vi "cam_track.vi"(6 "Trigger":bool, 7 "state change":bool, 8 "gun_rt_slow_downstream_data out in":T3, 9 "gun_rt_fast_downstream_data out":T4, 11 "Gains":T1) -> (2 "Lock":bool, 3 "gun_rt_slow_downstream_data out out":T3)   [LabVIEW 2011]
uses:
  gun_rt_slow_downstream_data.ctl
  gun_rt_fast_downstream_data.ctl
  gun_motor_state.ctl
  common/scale_const.ctl
  common/gain_bin_sched_const.ctl
  signals/Signal.ctl
  2012vision/Camera State.ctl
panel:
  in  "lock const":dbl=4.0
  in  "invert gains":bool
  out "settle time":dbl
  in  "Integral Cap":T2={"min_ana"=0.0, "min_units"=0.6, "max_ana"=0.4, "max_units"=0.0}
  in  "stop_track_time":u32=200
  in  "Cam Jitter Time":u32=500
  in  "Reset Integral":bool
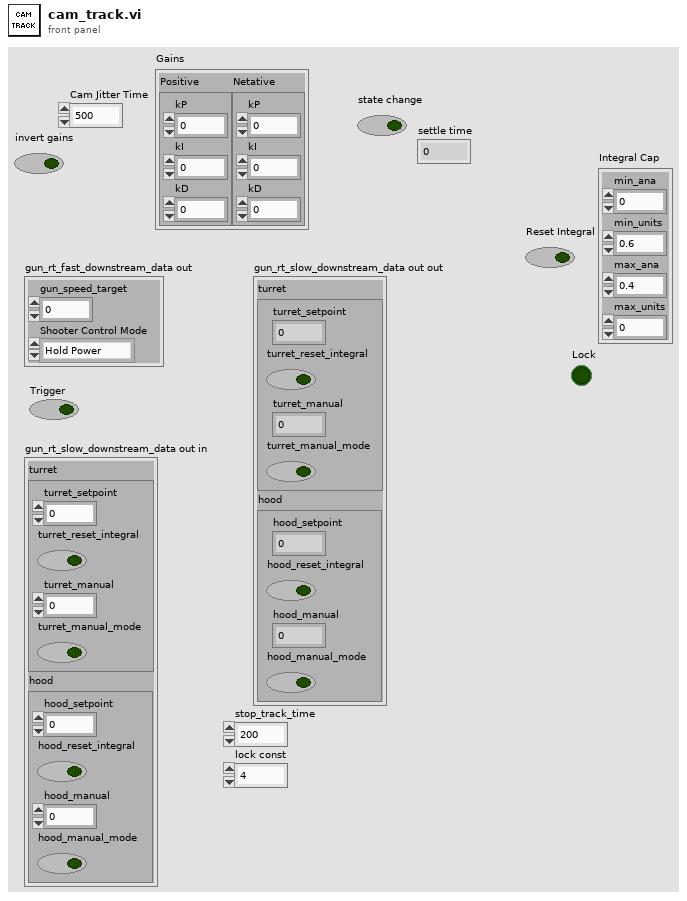
[diagram p1: front panel]
types:
  T1 = typedef "gain_bin_sched_const.ctl" = cluster{"Positive":cluster{"kP":dbl, "kI":dbl, "kD":dbl}, "Netative":cluster{"kP":dbl, "kI":dbl, "kD":dbl}}
  T2 = typedef "scale_const.ctl" = cluster{"min_ana":dbl, "min_units":dbl, "max_ana":dbl, "max_units":dbl}
  T3 = typedef "gun_rt_slow_downstream_data.ctl" = cluster{"turret":cluster{"turret_setpoint":dbl, "turret_reset_integral":bool, "turret_manual":dbl, "turret_manual_mode":bool}, "hood":cluster{"hood_setpoint":dbl, "hood_reset_integral":bool, "hood_manual":dbl, "hood_manual_mode":bool}}
  T4 = typedef "gun_rt_fast_downstream_data.ctl" = cluster{"gun_speed_target":dbl, "Shooter Control Mode":T5}
  T5 = typedef "gun_motor_state.ctl" = enum16{"Hold Power", "Hold Speed", "Hold Distance", "Stop"}
  T6 = typedef "Signal.ctl" = enum16{"SIGFIRE", "SIGSTOPSCRIPT", "SIGSTARTGUN", "SIGSTOPGUN", "SIGDISABLED", "SIGENABLED", "SIGUDPTIMEOUT", "SIGNEWVISION_REMOTE", "SIGNEWVISION_LOCAL", "SIGSHOTFIRED", "SIGDOTRACK", "SIGDONTTRACK"}
  T7 = typedef "Camera State.ctl" = enum16{"No Targets", "Low Confidence", "Medium Confidence", "High Confidence", "Camera Error"}
  T8 = enum16{"Get Latest Data", "Get Local Data", "Get Remote Data", "Set Local Data", "Set Remote Data"}
  T9 = cluster{"X Position":dbl, "Distance":dbl, "Camera State":T7}
  T10 = typedef "gain_const.ctl" = cluster{"kP":dbl, "kI":dbl, "kD":dbl}
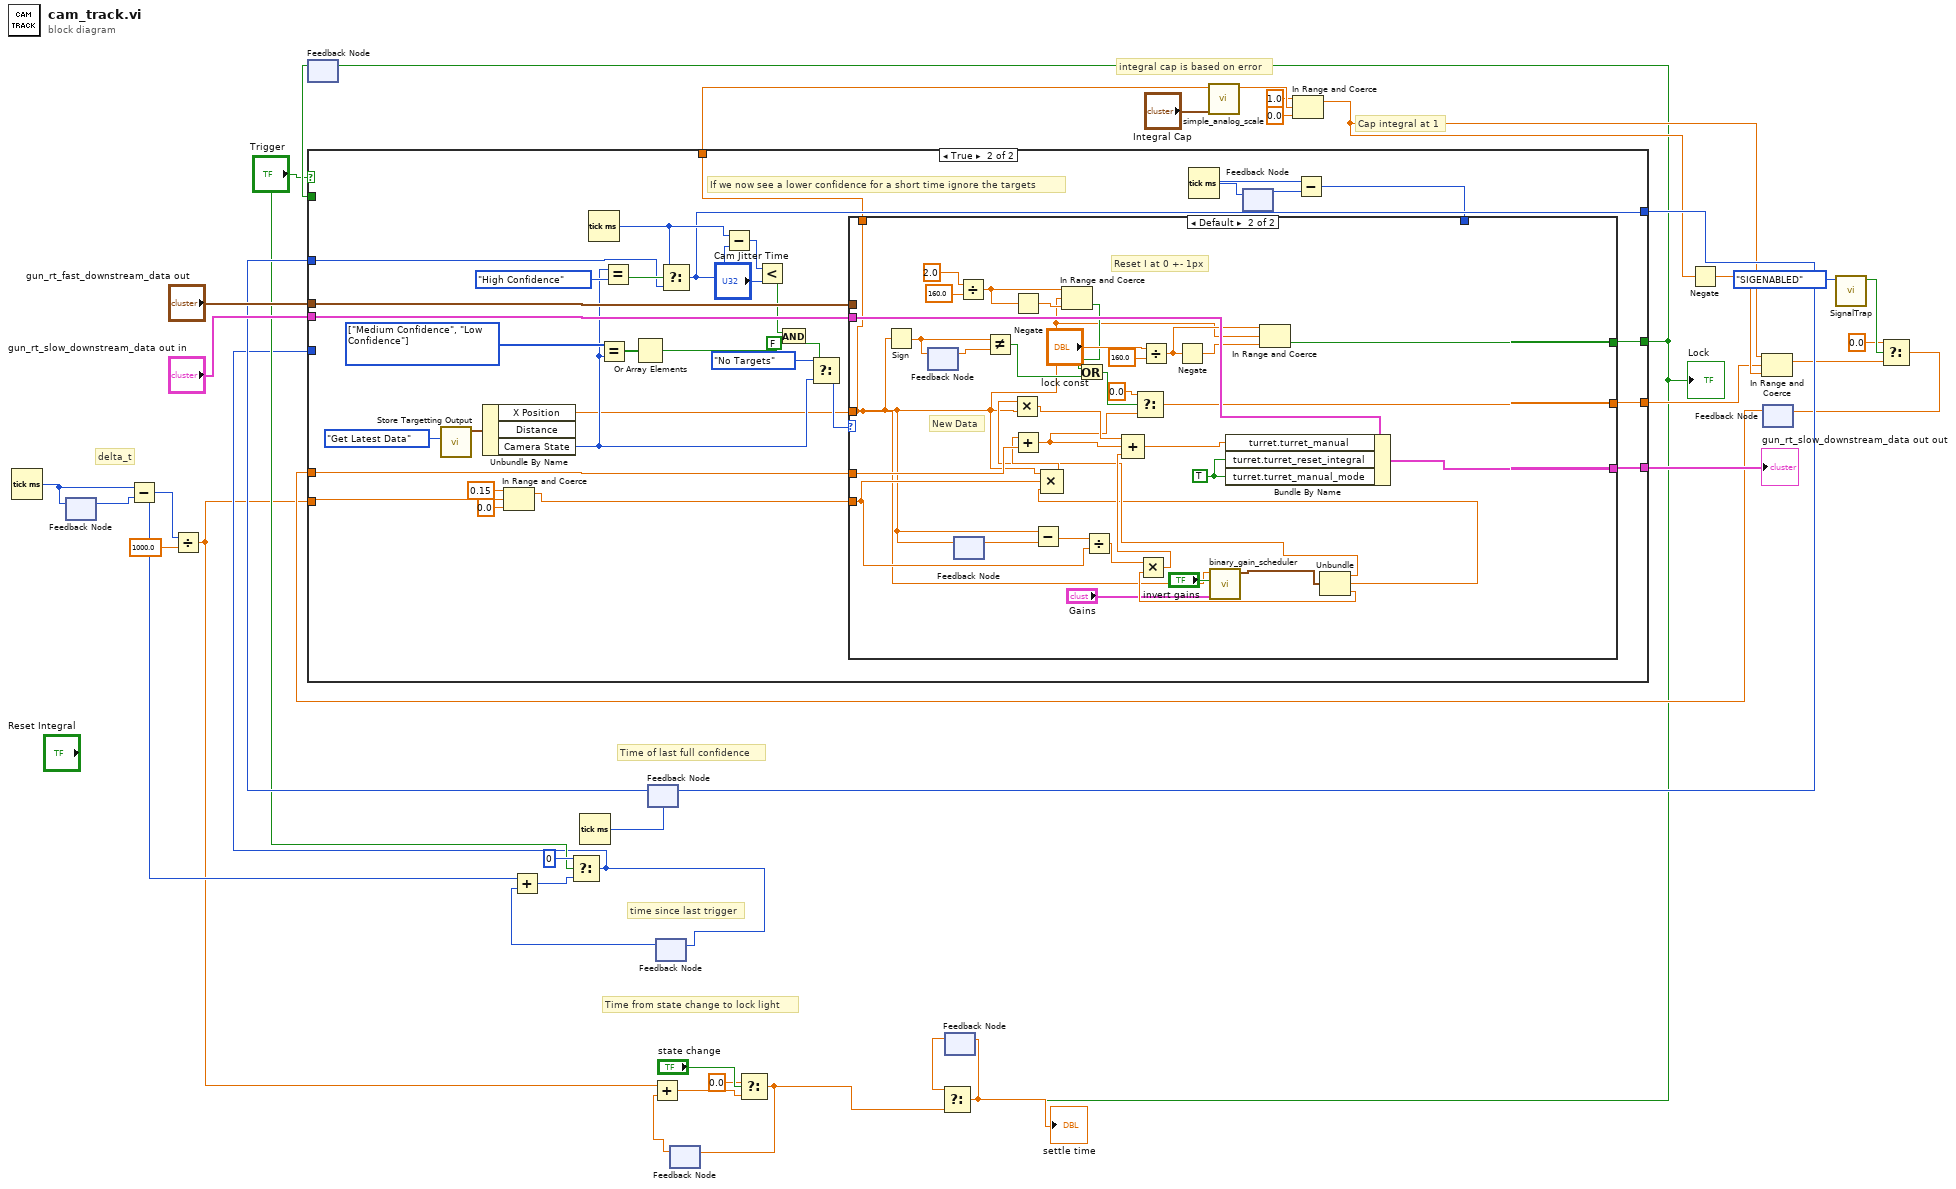
[diagram p0: block diagram]
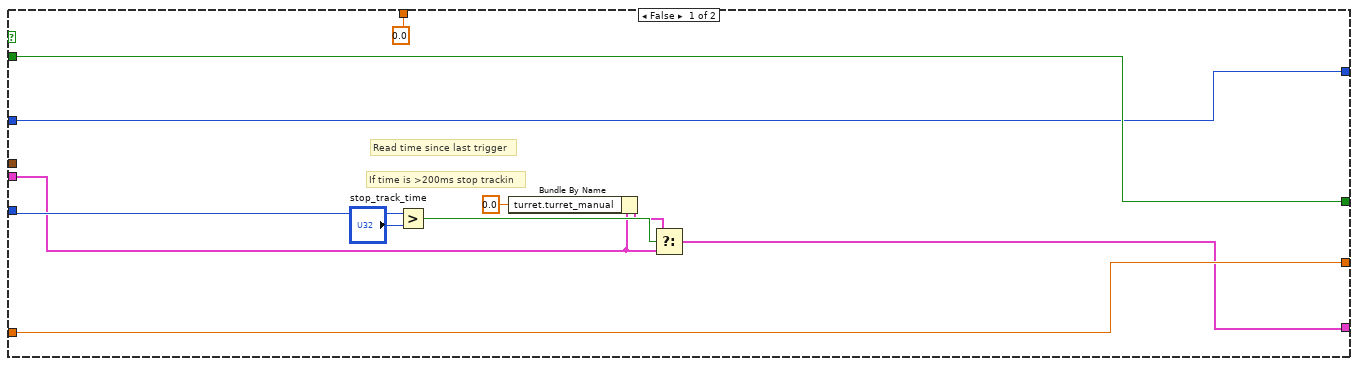
[diagram p2: hidden frame]
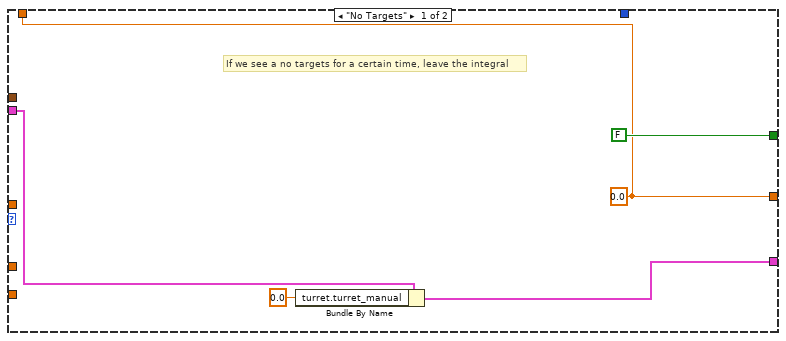
[diagram p3: hidden frame]
diagram:
  # "Time from state change to lock light"
  # "integral cap is based on error"
  # "time since last trigger"
  # "delta_t"
  # "Time of last full confidence"
  # "Cap integral at 1"
  n1 = Tick Count (ms)() -> (millisecond timer value=w30:u32)
  n2 = feedback-in #1(w30) -> ()
  n3 = feedback #1() -> (w29:u32)  [unwired: 1 in]
  n4 = Subtract(x=w30, y=w29) -> (x-y=w15:u32)
  n5 = Divide(x=w15, y=1000.0) -> (x/y=w9:dbl)
  n6 = feedback #2() -> (w36:bool)  [unwired: 1 in]
  n7 = Tick Count (ms)() -> (millisecond timer value=w33:u32)
  n8 = feedback #3(w33) -> (w32:u32)
  n9 = feedback #4() -> (w28:u32)  [unwired: 1 in]
  n10 = Add(x=w15, y=w28) -> (x+y=w27:u32)
  n11 = Select(t=u32 0, s="Trigger", f=w27) -> (s? t:f=w24:u32)
  n12 = feedback-in #4(w24) -> ()
  n13 = feedback #5() -> (w14:dbl)  [unwired: 1 in]
  n14 = Add(x=w9, y=w14) -> (x+y=w13:dbl)
  n15 = Select(t=0.0, s="state change", f=w13) -> (s? t:f=w1:dbl)
  n16 = feedback-in #5(w1) -> ()
  n17 = feedback #6() -> (w2:dbl)  [unwired: 1 in]
  n18 = feedback #7() -> (w35:dbl)  [unwired: 1 in]
  n19 = case shown="True" "Trigger" {
    tunnel: "gun_rt_slow_downstream_data out in" -> [w42 w80]
    tunnel: "gun_rt_fast_downstream_data out" -> [_ w79]
    tunnel: [w44 w78] -> w39
    tunnel: w36 -> [w50 _]
    tunnel: [w50 w77] -> w3
    tunnel: w35 -> [w49 w75]
    tunnel: [w49 w76] -> w16
    tunnel: w32 -> [w48 w72]
    tunnel: [w48 w67] -> w31
    tunnel: w24 -> [w47 _]
    tunnel: w9 -> [_ w57]
    tunnel: [0.0 ("X Position") w59] -> w22
    frame False {
      # "If time is >200ms stop trackin"
      # "Read time since last trigger"
      n20 = Greater?(x=w47, y="stop_track_time") -> (0:w45:bool)
      n21 = Bundle By Name(cluster=w42, "turret.turret_manual"=0.0) -> (w43:T3)
      n22 = Select(t=w43, s=w45, f=w42) -> (s? t:f=w44:T3)
    }
    frame True {
      w71 = T7[] [enum."Medium Confidence", enum."Low Confidence"] items=["No Targets", "Low Confidence", "Medium Confidence", "High Confidence", "Camera Error"]
      # "If we now see a lower confidence for a short time ignore the targets"
      n23 = call "Store Targetting Output.vi"("mode"=T8."Get Latest Data") -> ("Targetting Output"=w81:T9)  [unwired: 10 in]
      n24 = Unbundle By Name(w81) -> ("X Position"=w60:dbl, "Camera State"=w63:T7)  [unwired: 1 out]
      n25 = In Range and Coerce(upper limit=0.15, x=w57, lower limit=0.0) -> (coerced(x)=w55:dbl)  [unwired: 1 out]
      n26 = Tick Count (ms)() -> (millisecond timer value=w68:u32)
      n27 = Equal?(x=w71, y=w63) -> (x = y?=w70:bool[])
      n28 = Equal?(x=w63, y=Camera_State."High Confidence") -> (x = y?=w73:bool)
      n29 = Or Array Elements(Boolean array=w70) -> (logical OR=w69:bool)
      n30 = Select(t=w68, s=w73, f=w72) -> (s? t:f=w67:u32)
      n31 = Subtract(x=w68, y=w67) -> (x-y=w66:u32)
      n32 = Less?(x=w66, y="Cam Jitter Time") -> (x < y?=w64:bool)
      n33 = And(x=w64, y=w69) -> ()  [unwired: 1 out]
      n34 = Select(t=Camera_State."No Targets", s=FALSE, f=w63) -> (s? t:f=w62:T7)
      n35 = Tick Count (ms)() -> (millisecond timer value=w53:u32)
      n36 = feedback-in #8(w53) -> ()
      n37 = feedback #8() -> (w52:u32)  [unwired: 1 in]
      n38 = Subtract(x=w53, y=w52) -> (x-y=w51:u32)
      n39 = case shown="Default" w62 {
        tunnel: w60 -> [_ w88]
        tunnel: w80 -> [w86 w123]
        tunnel: w79 -> [_ _]
        tunnel: [w85 w122] -> w78
        tunnel: [FALSE w120] -> w77
        tunnel: [w83 w109] -> w76
        tunnel: w75 -> [_ w115]
        tunnel: w55 -> [_ w100]
        tunnel: [w83 w88] -> w59
        tunnel: w51 -> [_ _]
        frame "No Targets" {
          w83 = 0.0
          # "If we see a no targets for a certain time, leave the integral"
          n40 = Bundle By Name(cluster=w86, "turret.turret_manual"=0.0) -> (w85:T3)
        }
        frame Default {
          w121 = TRUE ("turret.turret_reset_integral")
          # "Reset I at 0 +- 1px"
          # "New Data"
          n41 = Sign(1:w88) -> (0:w105:dbl)
          n42 = feedback-in #9(w105) -> ()
          n43 = feedback #9() -> (w104:dbl)  [unwired: 1 in]
          n44 = feedback-in #10(w88) -> ()
          n45 = feedback #10() -> (w102:dbl)  [unwired: 1 in]
          n46 = Divide(x=2.0, y=160.0) -> (x/y=w110:dbl)
          n47 = Not Equal?(x=w105, y=w104) -> (x != y?=w103:bool)
          n48 = Negate(x=w110) -> (-x=w111:dbl)
          n49 = Subtract(x=w88, y=w102) -> (x-y=w101:dbl)
          n50 = In Range and Coerce(upper limit=w110, x=w88, lower limit=w111) -> (In Range?=w106:bool)  [unwired: 1 out]
          n51 = Or(x=w106, y=w103) -> (x .or. y?=w95:bool)
          n52 = Divide(x=w101, y=w100) -> (x/y=w99:dbl)
          n53 = Divide(x="lock const", y=160.0) -> (x/y=w116:dbl)
          n54 = Negate(x=w116) -> (-x=w117:dbl)
          n55 = call "binary_gain_scheduler.vi"("Binary scheduling constant"="Gains", "Invert"="invert gains", "Error"=w88) -> ("Gains out"=w91:T10)  [unwired: 8 in]
          n56 = In Range and Coerce(upper limit=w116, x=w88, lower limit=w117) -> (In Range?=w120:bool)  [unwired: 1 out]
          n57 = Unbundle(w91) -> ("kP"=w94:dbl, "kI"=w93:dbl, "kD"=w92:dbl)
          n58 = Multiply(x=w94, y=w88) -> (x*y=w107:dbl)
          n59 = Compound Arithmetic op=MULTIPLY(w88, w100, w93) -> (w97:dbl)
          n60 = Add(x=w97, y=w115) -> (x+y=w96:dbl)
          n61 = Select(t=0.0, s=w95, f=w96) -> (s? t:f=w109:dbl)
          n62 = Multiply(x=w99, y=w92) -> (x*y=w98:dbl)
          n63 = Compound Arithmetic op=ADD(w107, w96, w98) -> (w114:dbl)
          n64 = Bundle By Name(cluster=w123, "turret.turret_manual"=w114, "turret.turret_reset_integral"=w121, "turret.turret_manual_mode"=w121) -> (w122:T3)
        }
      }
    }
  }
  "gun_rt_slow_downstream_data out out" <- w39
  "Lock" <- w3
  n65 = feedback-in #2(w3) -> ()
  n66 = feedback-in #3(w31) -> ()
  n67 = Select(t=w2, s=w3, f=w1) -> (s? t:f=w10:dbl)
  "settle time" <- w10
  n68 = feedback-in #6(w10) -> ()
  n69 = call "simple_analog_scale.vi"("Scale Const"="Integral Cap", "Analog"=w22) -> ("Units"=w20:dbl)  [unwired: 9 in]
  n70 = In Range and Coerce(upper limit=1.0, x=w20, lower limit=0.0) -> (coerced(x)=w19:dbl)  [unwired: 1 out]
  n71 = Negate(x=w19) -> (-x=w34:dbl)
  n72 = In Range and Coerce(upper limit=w19, x=w16, lower limit=w34) -> (coerced(x)=w7:dbl)  [unwired: 1 out]
  n73 = call "SignalTrap.vi"("Signal"=Signal."SIGENABLED") -> ("Trapped Signal"=w5:bool)  [unwired: 10 in]
  n74 = Select(t=0.0, s=w5, f=w7) -> (s? t:f=w6:dbl)
  n75 = feedback-in #7(w6) -> ()
